vi "open_visa_resources.vi"(7 "test mode":bool, 8 "error in (no error)":errorcluster, 11 "config file in":string="VISA_config.ini") -> (0 "error out":errorcluster, 2 "Assgs":T2, 3 "VISA":T1)   [LabVIEW 2015]
uses:
  Type Definitions/get_visa_resources_states.ctl
  Type Definitions/get_visa_resources_data.ctl
panel:
  # "NOTE: There are only two\ntest modes: \ntest_mode=FALSE, GB test then \nHi-Pot test\ntest_mode=TRUE, Hi-Pot test only"
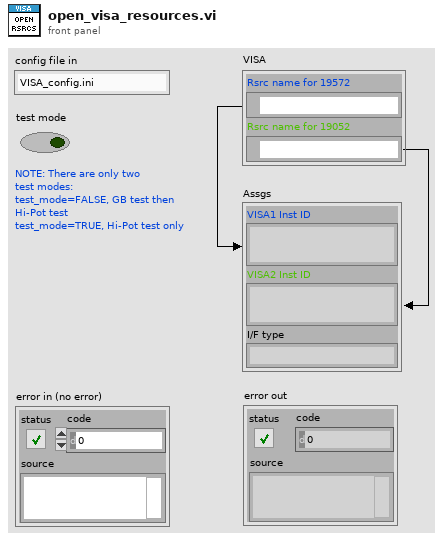
[diagram p1: front panel]
types:
  T1 = cluster{"Rsrc name for 19572":refnum<visa-resource-name>, "Rsrc name for 19052":refnum<visa-resource-name>}
  T2 = cluster{"VISA1 Inst ID":string, "VISA2 Inst ID":string, "I/F type":string}
  T3 = typedef "get_visa_resources_data.ctl" = cluster{"Test mode":bool, "19052 COM":cluster{"COM port":string, "b rate":string, "f control":string, "parity":string}, "19572 COM":cluster{"COM port":string, "b rate":string, "f control":string, "parity":string}, "Assgs":cluster{"VISA1 Inst ID":string, "VISA2 Inst ID":string, "I/F type":string}}
  T4 = typedef "get_visa_resources_states.ctl" = enum16{"Initialize", "Get Interface type", "Build VISA Rsrc Name (GPIB)", "Build VISA Rsrc Name (RS232)", "Set RS232 parameters", "Get Instrument ID(s)", "Shutdown"}
  T5 = cluster{"gpib_board_No.":string, "19572_gpib_prim_adr":string, "19052_gpib_prim_adr":string}
  T6 = cluster{"COM port":string, "baud rate":string, "flow control":string, "parity":string}
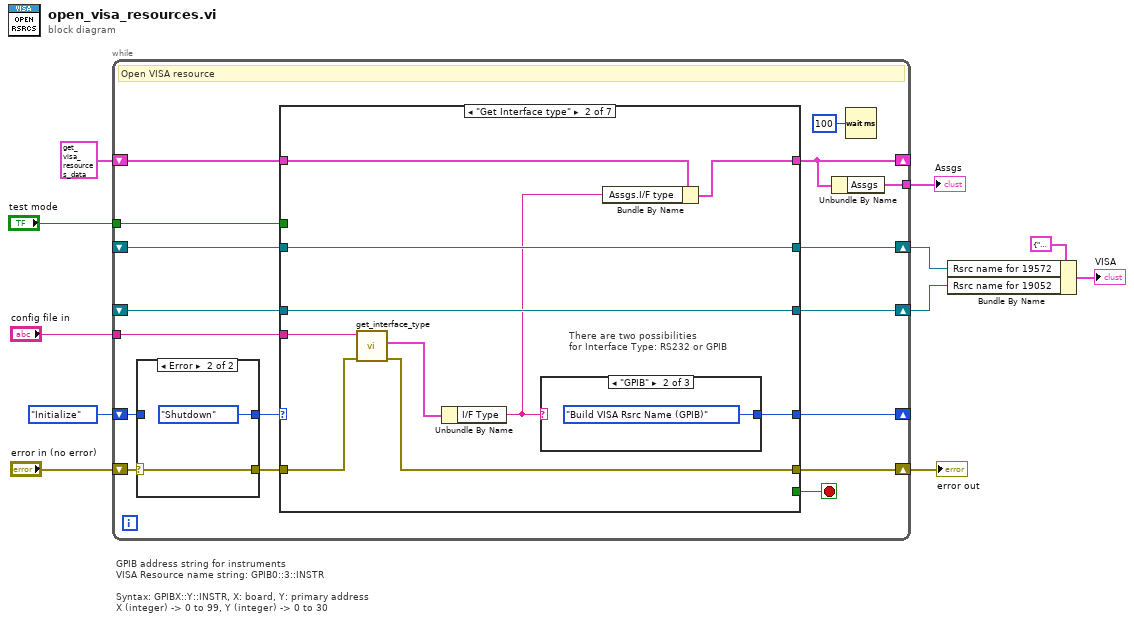
[diagram p0: block diagram]
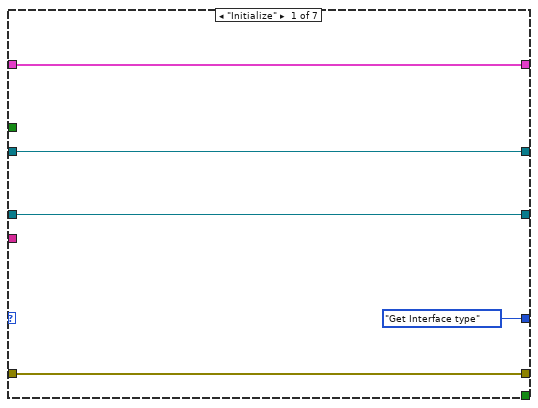
[diagram p3: hidden frame]
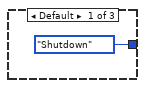
[diagram p4: hidden frame]
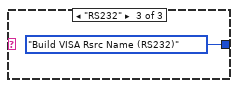
[diagram p5: hidden frame]
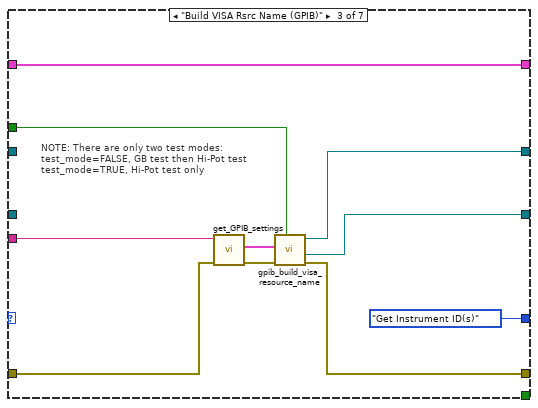
[diagram p6: hidden frame]
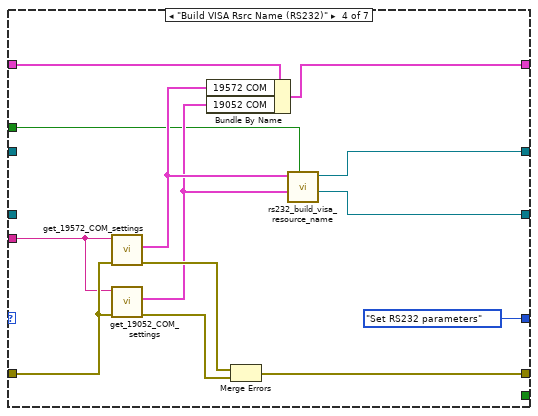
[diagram p7: hidden frame]
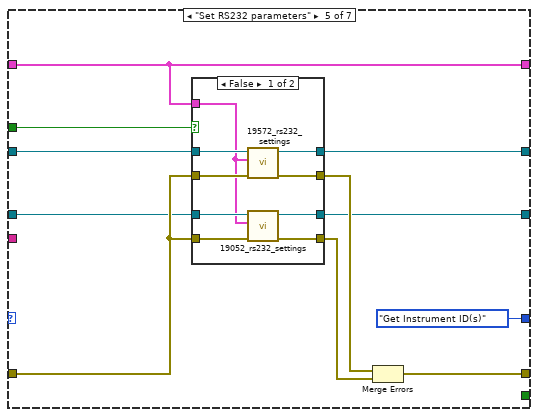
[diagram p8: hidden frame]
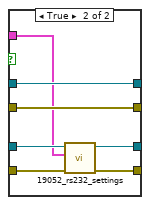
[diagram p9: hidden frame]
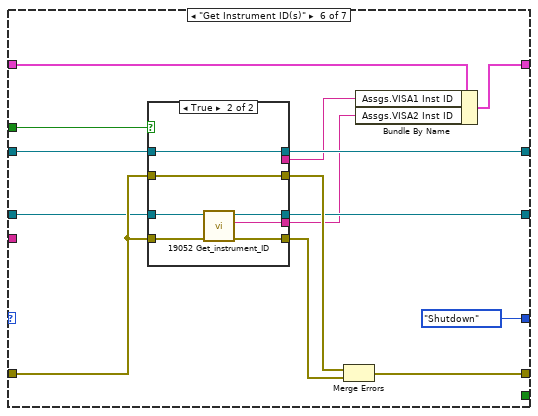
[diagram p10: hidden frame]
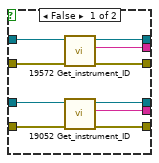
[diagram p11: hidden frame]
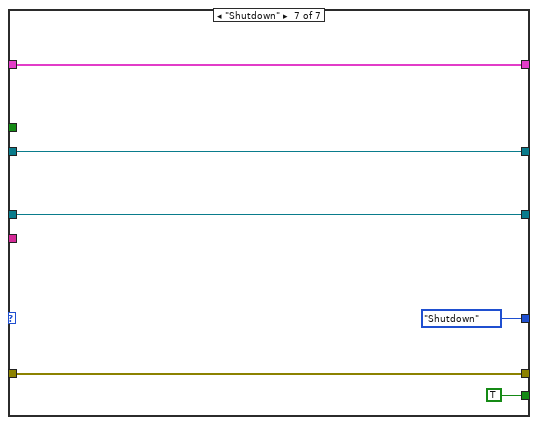
[diagram p12: hidden frame]
diagram:
  # "GPIB address string for instruments\nVISA Resource name string: GPIB0::3::INSTR\n\nSyntax: GPIBX::Y::INSTR, X: board, Y: primary address\nX (integer) -> 0 to 99, Y (integer) -> 0 to 30"
  n1 = while {
    shift-right: [w26] -> w10
    shift-left: "error in (no error)" -> [w28]
    shift-right: [w23] -> _
    shift-left: get_visa_resources_states."Initialize" -> [w25]
    tunnel: "test mode" -> [w21]
    shift-right: [w18] -> _
    shift-left: T3 {"Test mode"=TRUE, "19052 COM"={"COM port"="", "b rate"="", "f control"="", "parity"=""}, "19572 COM"={"COM port"="", "b rate"="", "f control"="", "parity"=""}, "Assgs"={"VISA1 Inst ID"="", "VISA2 Inst ID"="", "I/F type"=""}} -> [w20]
    tunnel: "config file in" -> [w19]
    tunnel: [w16] -> w5
    shift-right: [w15] -> w4
    shift-left: _ -> [w13]
    shift-right: [w14] -> w3
    shift-left: _ -> [w12]
    stop <- w22 stop-if-true
    # "Open VISA resource"
    n2 = case shown="Error" w28 {
      selector: w28 -> [w30 w32]
      tunnel: [w30 w32] -> w27
      tunnel: w25 -> [w29 _]
      tunnel: [w29 get_visa_resources_states."Shutdown"] -> w24
      frame No Error {
      }
      frame Error {
      }
    }
    n3 = case shown="\"Get Interface type\"" w24 {
      tunnel: w27 -> [w37 w46 w59 w71 w83 w114 w137]
      tunnel: [w37 w45 w57 w61 w80 w103 w137] -> w26
      tunnel: [get_visa_resources_states."Get Interface type" w44 get_visa_resources_states."Get Instrument ID(s)" get_visa_resources_states."Set RS232 parameters" get_visa_resources_states."Get Instrument ID(s)" get_visa_resources_states."Shutdown" get_visa_resources_states."Shutdown"] -> w23
      tunnel: [_ _ _ _ _ _ TRUE] -> w22
      tunnel: w21 -> [_ _ w55 w63 w81 w111 _]
      tunnel: w20 -> [w36 w43 w53 w72 w75 w101 w136]
      tunnel: [w36 w42 w53 w69 w75 w110 w136] -> w18
      tunnel: w19 -> [_ w47 w60 w67 _ _ _]
      tunnel: [w34 w41 w54 w68 w78 w106 w133] -> w15
      tunnel: [w33 w40 w52 w64 w76 w105 w132] -> w14
      tunnel: w13 -> [w34 w41 _ _ w79 w108 w133]
      tunnel: w12 -> [w33 w40 _ _ w77 w107 w132]
      frame "Initialize" {
      }
      frame "Get Interface type" {
        # "There are two possibilities\nfor Interface Type: RS232 or GPIB"
        n4 = call "get_interface_type.vi"("error in (no error)"=w46, "config_file_name"=w47) -> ("error out"=w45:errorcluster, "Data"=w39:cluster{"I/F Type":string})  [unwired: 7 in, 1 out]
        n5 = Unbundle By Name(w39) -> ("I/F Type"=w38:string)
        n6 = case shown="\"GPIB\"" w38 {
          tunnel: [get_visa_resources_states."Shutdown" get_visa_resources_states."Build VISA Rsrc Name (GPIB)" get_visa_resources_states."Build VISA Rsrc Name (RS232)"] -> w44
          frame Default {
          }
          frame "GPIB" {
          }
          frame "RS232" {
          }
        }
        n7 = Bundle By Name(cluster=w43, "Assgs.I/F type"=w38) -> (w42:T3)
      }
      frame "Build VISA Rsrc Name (GPIB)" {
        # "NOTE: There are only two test modes: \ntest_mode=FALSE, GB test then Hi-Pot test\ntest_mode=TRUE, Hi-Pot test only"
        n8 = call "get_GPIB_settings.vi"("error in (no error)"=w59, "config_file_name"=w60) -> ("error out"=w58:errorcluster, "GPIB settings"=w56:T5)  [unwired: 7 in, 1 out]
        n9 = call "gpib_build_visa_resource_name.vi"("test mode"=w55, "error in (no error)"=w58, "GPIB settings"=w56) -> ("error out"=w57:errorcluster, "VISA Resource name 2"=w52:refnum<visa-resource-name>, "VISA Resource name 1"=w54:refnum<visa-resource-name>)  [unwired: 6 in]
      }
      frame "Build VISA Rsrc Name (RS232)" {
        n10 = call "get_19572_COM_settings.vi"("error in (no error)"=w71, "config_file_name"=w67) -> ("error out"=w66:errorcluster, "19572 COM settings"=w73:T6)  [unwired: 7 in, 1 out]
        n11 = call "get_19052_COM_settings.vi"("error in (no error)"=w71, "config_file_name"=w67) -> ("error out"=w70:errorcluster, "19052 COM settings"=w65:T6)  [unwired: 7 in, 1 out]
        n12 = Bundle By Name(cluster=w72, "19572 COM"=w73, "19052 COM"=w65) -> (w69:T3)
        n13 = Merge Errors(w66, w70) -> (w61:errorcluster)
        n14 = call "rs232_build_visa_resource_name.vi"("test mode"=w63, "19052 COM settings"=w65, "19572 COM settings"=w73) -> ("VISA Resource name 2"=w64:refnum<visa-resource-name>, "VISA Resource name 1"=w68:refnum<visa-resource-name>)  [unwired: 7 in]
      }
      frame "Set RS232 parameters" {
        n15 = case shown="False" w81 {
          tunnel: [w93 w100] -> w82
          tunnel: w75 -> [w85 w94]
          tunnel: [w92 w99] -> w84
          tunnel: w83 -> [w87 w95]
          tunnel: w79 -> [w89 w98]
          tunnel: [w91 w98] -> w78
          tunnel: w77 -> [w86 w96]
          tunnel: [w90 w97] -> w76
          tunnel: w83 -> [w88 w100]
          frame False {
            n16 = call "19572_rs232_settings.vi"("error in (no error)"=w88, "input cluster"=w85, "reference in"=w89) -> ("error out"=w93:errorcluster, "reference out"=w91:refnum<visa-resource-name>)  [unwired: 7 in]
            n17 = call "19052_rs232_settings.vi"("error in (no error)"=w87, "input cluster"=w85, "reference in"=w86) -> ("error out"=w92:errorcluster, "reference out"=w90:refnum<visa-resource-name>)  [unwired: 7 in]
          }
          frame True {
            n18 = call "19052_rs232_settings.vi"("error in (no error)"=w95, "input cluster"=w94, "reference in"=w96) -> ("error out"=w99:errorcluster, "reference out"=w97:refnum<visa-resource-name>)  [unwired: 7 in]
          }
        }
        n19 = Merge Errors(w82, w84) -> (w80:errorcluster)
      }
      frame "Get Instrument ID(s)" {
        n20 = case shown="True" w111 {
          tunnel: w108 -> [w124 w128]
          tunnel: w107 -> [w122 w131]
          tunnel: [w123 _] -> w104
          tunnel: [w119 w130] -> w102
          tunnel: [w121 w128] -> w106
          tunnel: [w120 w129] -> w105
          tunnel: w114 -> [w118 w125]
          tunnel: w114 -> [w117 w127]
          tunnel: [w116 w125] -> w113
          tunnel: [w115 w126] -> w112
          frame False {
            n21 = call "19572 Get_instrument_ID.vi"("error in"=w118, "VISA resource name in"=w124) -> ("error out"=w116:errorcluster, "instrument ID"=w123:string, "VISA resource name out"=w121:refnum<visa-resource-name>)  [unwired: 7 in]
            n22 = call "19052 Get_instrument_ID.vi"("error in"=w117, "VISA resource name in"=w122) -> ("error out"=w115:errorcluster, "instrument ID"=w119:string, "VISA resource name out"=w120:refnum<visa-resource-name>)  [unwired: 7 in]
          }
          frame True {
            n23 = call "19052 Get_instrument_ID.vi"("error in"=w127, "VISA resource name in"=w131) -> ("error out"=w126:errorcluster, "instrument ID"=w130:string, "VISA resource name out"=w129:refnum<visa-resource-name>)  [unwired: 7 in]
          }
        }
        n24 = Merge Errors(w113, w112) -> (w103:errorcluster)
        n25 = Bundle By Name(cluster=w101, "Assgs.VISA1 Inst ID"=w104, "Assgs.VISA2 Inst ID"=w102) -> (w110:T3)
      }
      frame "Shutdown" {
      }
    }
    n26 = Unbundle By Name(w18) -> ("Assgs"=w16:T2)
    n27 = Wait (ms)(milliseconds to wait=u32 100) -> ()  [unwired: 1 out]
  }
  "error out" <- w10
  "Assgs" <- w5
  n28 = Bundle By Name(cluster=T1 {"Rsrc name for 19572"="ASRL6::INSTR", "Rsrc name for 19052"="ASRL5::INSTR"} ("VISA"), "Rsrc name for 19572"=w4, "Rsrc name for 19052"=w3) -> (→"VISA":T1)
